vi "LoadServerCfg.vi"(8 "error in (no error)":errorcluster, 11 "RESTLoaderBase in":refnum<class "RESTLoaderBase.lvclass">) -> (0 "error out":errorcluster, 2 "Server config":T1={"API Root"="", "verify server"=FALSE, "Version (no version)"="", "Port (protocol specific)"=0, "Base URL"="", "Auth type"=enum."Token", "Auth string"="", "timeout (10000)"=10000}, 3 "RESTLoaderBase out":refnum<class "RESTLoaderBase.lvclass">)   [LabVIEW 2019, in "ByteREST.lvlib" / "RESTLoaderBase.lvclass"]
uses:
  RESTLoaderBase.lvclass
  ServerParams.ctl
  ByteRESTClass/ByteRESTBase/Auth/Authentication_type.ctl
  ByteRESTClass/ByteRESTBase/RESTBase.lvclass
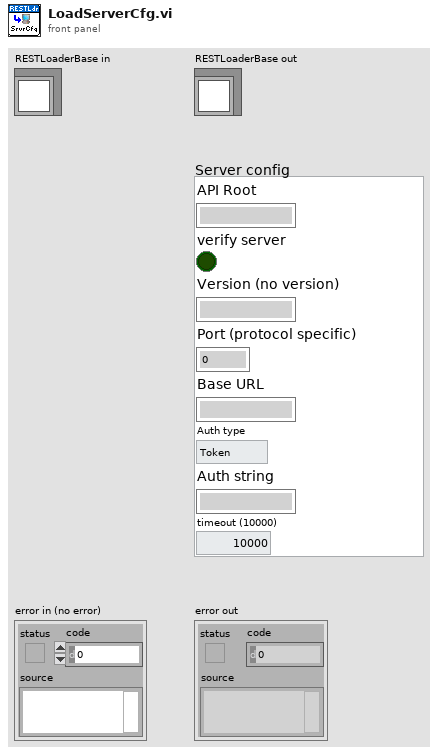
[diagram p1: front panel]
types:
  T1 = typedef "ServerParams.ctl" = cluster{"API Root":string, "verify server":bool, "Version (no version)":string, "Port (protocol specific)":u16, "Base URL":string, "Auth type":T2, "Auth string":string, "timeout (10000)":i32}
  T2 = typedef "ByteREST.lvlib/RESTBase.lvclass/Authentication_type.ctl" = enum16{"Token"}
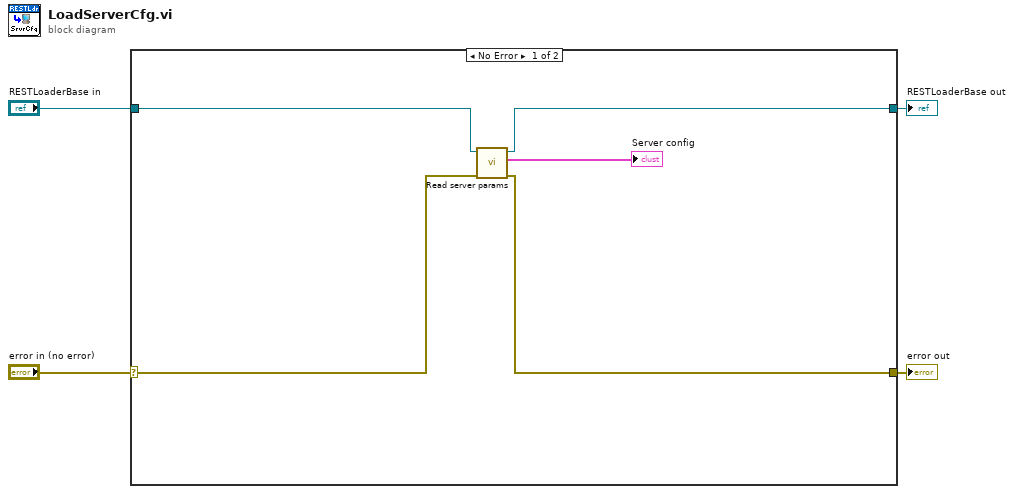
[diagram p0: block diagram]
diagram:
  n1 = case shown="No Error" "error in (no error)" {
    selector: "error in (no error)" -> [w6 w11]
    tunnel: [w5 w11] -> w3
    tunnel: [w8 w10] -> w1
    tunnel: "RESTLoaderBase in" -> [w9 w10]
    frame No Error {
      n2 = call "Read server params.vi"("error in (no error)"=w6, "RESTLoaderBase in"=w9) -> ("error out"=w5:errorcluster, "Server config"=→"Server config":T1, "RESTLoaderBase out"=w8:refnum<class "RESTLoaderBase.lvclass">)  [unwired: 7 in]
    }
    frame Error {
    }
  }
  "error out" <- w3
  "RESTLoaderBase out" <- w1
